vi "Com_SECS Equipment _Build SECS Packet.vi"(7 "Build Message Setting":T1, 8 "error in":errorcluster, 11 "Message Data":T2[](array[typedef])) -> (0 "error out":errorcluster, 3 "SECS Packet":T5)   [LabVIEW 2016]
uses:
  Data Def/Com_SECS Equipment _SECS Packet.ctl
  Data Def/Com_SECS Equipment _Message Type.ctl
  Data Def/Com_SECS Equipment _Protocol Type.ctl
  Data Def/Com_SECS Equipment _Stream Type.ctl
  Data Def/Com_SECS Equipment _Message Data.ctl
  Data Def/Com_SECS Equipment _Data Item Format.ctl
  Data Def/Com_SECS Equipment _Format Code.ctl
  Data Def/Com_SECS Equipment _Build Message Setting.ctl
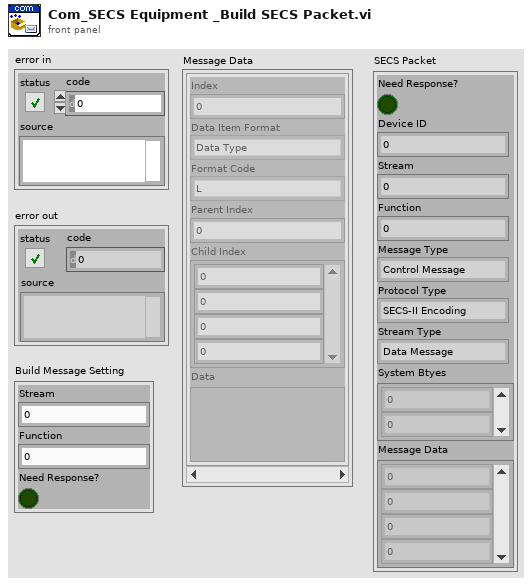
[diagram p1: front panel]
types:
  T1 = typedef "Com_SECS Equipment _Build Message Setting.ctl" = cluster{"Stream":u8, "Function":u8, "Need Response?":bool}
  T2 = typedef "Com_SECS Equipment _Message Data.ctl" = cluster{"Index":i32, "Data Item Format":T3, "Format Code":T4, "Parent Index":i32, "Child Index":i32[], "Data":variant}
  T3 = typedef "Com_SECS Equipment _Data Item Format.ctl" = enum16{"Data Type", "Value"}
  T4 = typedef "Com_SECS Equipment _Format Code.ctl" = enum16{"L", "A", "B", "Boolean", "J", "I1", "I2", "I4", "I8", "U1", "U2", "U4", "U8", "F4", "F8", "Char"}
  T5 = typedef "Com_SECS Equipment _SECS Packet.ctl" = cluster{"Need Response?":bool, "Device ID":u16, "Stream":u8, "Function":u8, "Message Type":T6, "Protocol Type":T7, "Stream Type":T8, "System Btyes":u8[], "Message Data":u8[]}
  T6 = typedef "Com_SECS Equipment _Message Type.ctl" = enum16{"Control Message", "Data Message"}
  T7 = typedef "Com_SECS Equipment _Protocol Type.ctl" = enum16{"SECS-II Encoding", "Reserved"}
  T8 = typedef "Com_SECS Equipment _Stream Type.ctl" = enum16{"Data Message", "Select.req", "Select.rsp", "Deselect.req", "Deselect.rsp", "Linktest.req", "Linktest.rsp", "Reject.req", "Separate.req", "Reserve"}
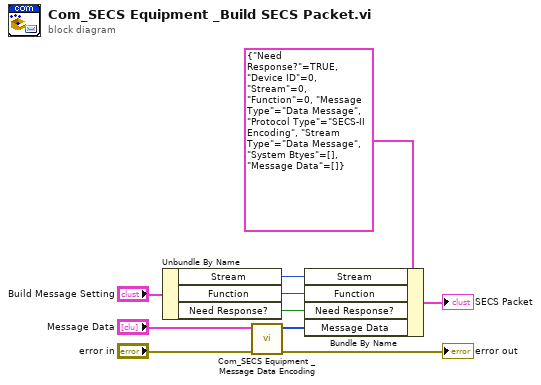
[diagram p0: block diagram]
diagram:
  n1 = Unbundle By Name("Build Message Setting") -> ("Stream"=w3:u8, "Function"=w2:u8, "Need Response?"=w1:bool)
  n2 = call "Com_SECS Equipment _Message Data Encoding.vi"("error in"="error in", "Message Data In"="Message Data") -> ("error out"=→"error out":errorcluster, "Message Data Out"=w7:u8[])  [unwired: 8 in]
  n3 = Bundle By Name(cluster=T5 {"Need Response?"=TRUE, "Device ID"=0, "Stream"=0, "Function"=0, "Message Type"=enum."Data Message", "Protocol Type"=enum."SECS-II Encoding", "Stream Type"=enum."Data Message", "System Btyes"=[], "Message Data"=[]} ("SECS Packet"), "Stream"=w3, "Function"=w2, "Need Response?"=w1, "Message Data"=w7) -> (→"SECS Packet":T5)
